vi "Initialize Front Panel.vi"(8 "error in (no error)":errorcluster, 11 "For Loop Dialog in":refnum<class "For Loop Dialog.lvclass">) -> (0 "error out":errorcluster, 3 "For Loop Dialog out":refnum<class "For Loop Dialog.lvclass">)   [LabVIEW 2017, in "For Loop Dialog.lvclass"]
doc: "<License>\nCopyright © 2017 Composed Systems, LLC | All rights reserved\nwww.composed.io\n\nAuthor: Ethan Stern <ethan.stern@composed.io>\n\nThis software is provided \"AS IS\" WITHOUT WARRANTIES, either express or implied, AND IS FOR EDUCATIONAL PURPOSES ONLY.\n</License>"
uses:
  <vilib>/gpm_packages/@cs/Test-executive-builder/Source/Test Executive Builder Dialogs/For Loop Dialog/For Loop Dialog.lvclass
  <vilib>/gpm_packages/@cs/Test-executive-builder/Source/Test Executive Builder Dialogs/For Loop Dialog/For Loop Dialog.lvclass/For Loop Dialog.ctl
  <vilib>/gpm_packages/@cs/Test-executive-builder/Source/Test Executive Builder Dialogs/ITest Executive Builder Dialog/ITest Executive Builder Dialog.lvclass
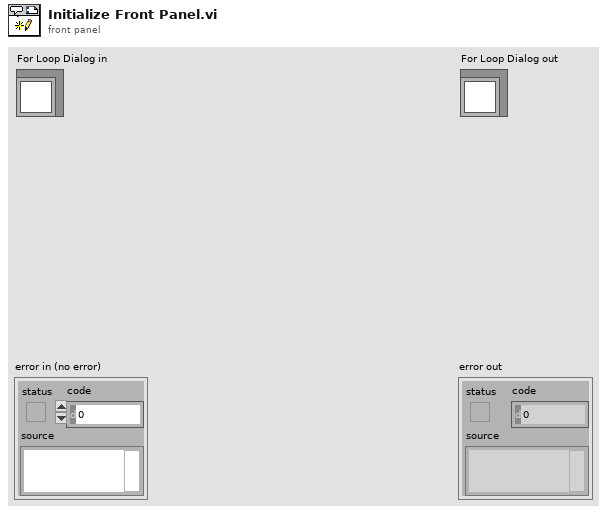
[diagram p1: front panel]
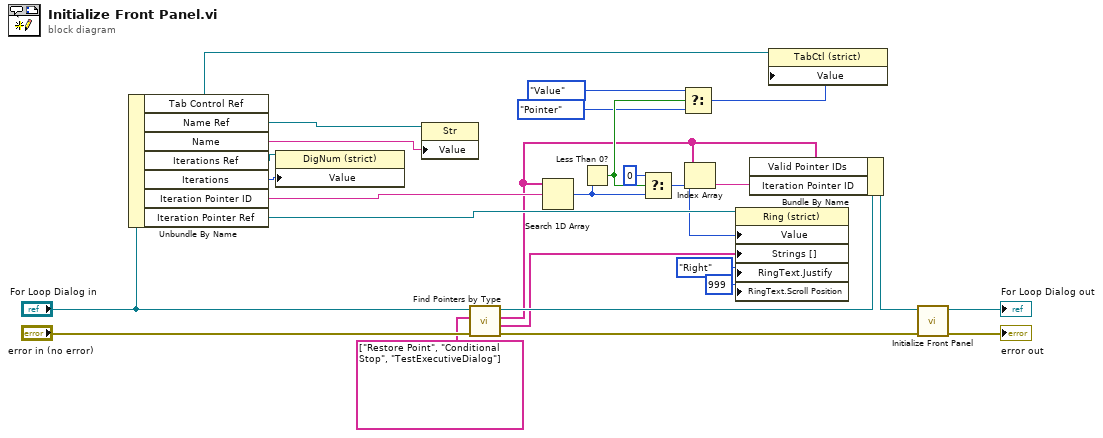
[diagram p0: block diagram]
diagram:
  n1 = Unbundle By Name("For Loop Dialog in") -> ("Tab Control Ref"=w12:refnum<vi>, "Name Ref"=w16:refnum<vi>, "Name"=w15:string, "Iterations Ref"=w14:refnum<vi>, "Iterations"=w13:u32, "Iteration Pointer ID"=w25:string, "Iteration Pointer Ref"=w20:refnum<vi>)
  n2 = property class="DigNum (strict)"(reference=w14, "Value"=w13) -> ()  [unwired: 1 in, 2 out]
  n3 = property class="Str"(reference=w16, "Value"=w15) -> ()  [unwired: 1 in, 2 out]
  n4 = call-dynamic "Find Pointers by Type.vi"("error in (no error)"="error in (no error)", "Exclusion List"=string[] ["Restore Point", "Conditional Stop", "TestExecutiveDialog"], "For Loop Dialog in"="For Loop Dialog in") -> ("error out"=w4:errorcluster, "Valid Pointer Names"=w2:string[], "Valid Pointer IDs"=w1:string[], "For Loop Dialog out"=w6:refnum<class "For Loop Dialog.lvclass">)  [unwired: 5 in]
  n5 = Search 1D Array(1D array=w1, element=w25) -> (index of element=w24:i32)  [unwired: 1 in]
  n6 = Less Than 0?(x=w24) -> (x < 0?=w11:bool)
  n7 = Select(t=0, s=w11, f=w24) -> (s? t:f=w19:i32)
  n8 = Select(t=enum32{"Value", "Pointer"}."Value" ("Value"), s=w11, f=enum32{"Value", "Pointer"}."Pointer" ("Value")) -> (s? t:f=w9:enum32{"Value", "Pointer"})
  n9 = Index Array(array=w1, index=w19) -> (element=w22:string)
  n10 = property class="Ring (strict)"(reference=w20, "Value"=w19, "Strings []"=w2, "RingText.Justify"=enum16{"Left", "Center", "Right"}."Right" ("Ring Text.Justification"), "RingText.Scroll Position"=u32 999 ("Ring Text.Scroll Position")) -> ()  [unwired: 1 in, 2 out]
  n11 = Bundle By Name(cluster=w6, "Valid Pointer IDs"=w1, "Iteration Pointer ID"=w22) -> (w21:refnum<class "For Loop Dialog.lvclass">)
  n12 = property class="TabCtl (strict)"(reference=w12, "Value"=w9) -> ()  [unwired: 1 in, 2 out]
  n13 = call-parent "Initialize Front Panel.vi"("error in (no error)"=w4, "ITest Executive Builder Dialog in"=w21) -> ("error out"=→"error out":errorcluster, "ITest Executive Builder Dialog out"=→"For Loop Dialog out":refnum<class "For Loop Dialog.lvclass">)  [unwired: 8 in]
